vi "Filter Reorder Denominator Coefficients to FPGA SOS Order.vi"(11 "coef a (k)":dbl[](array[numeric])) -> (3 "coef a (k)":dbl[](array[numeric]))   [LabVIEW 2011]
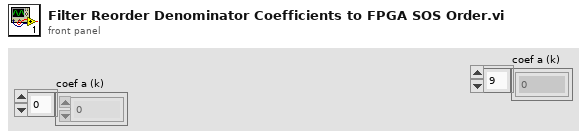
[diagram p1: front panel]
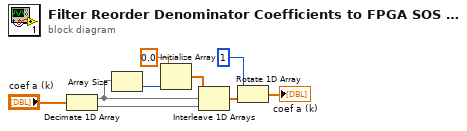
[diagram p0: block diagram]
diagram:
  n1 = Decimate 1D Array("coef a (k)") -> (w8:dbl[], w9:dbl[])
  n2 = Array Size(array=w8) -> (size(s)=w5:i32)
  n3 = Initialize Array(0.0 ("element"), w5) -> (w7:dbl[])
  n4 = Interleave 1D Arrays(w7, w8, w9) -> (w4:dbl[])
  n5 = Rotate 1D Array(1:w4, 2:1 ("n")) -> (0:→"coef a (k)":dbl[])
